vi "USRP_singlecarrierTDMUSRP1.vi"() -> ()   [LabVIEW 2021]
uses:
  <vilib>/addons/Modulation/Analog/controls/Complex Data Waveform.ctl
  <vilib>/Analysis/coordinate.llb/Angle Units.ctl
  <vilib>/Analysis/coordinate.llb/Angle Range (Degree).ctl
  <vilib>/Analysis/coordinate.llb/Wrap Angle (scalar).vi
  system stop.vi
  <vilib>/measure/matone.llb/Extract Single Tone Information 1 Chan (CDB).vi
  <instrlib>/niUSRP/niUSRP Fetch Rx Data (CDB Cluster).vi
  <instrlib>/niUSRP/niUSRP Write Tx Data (CDB Cluster).vi
  <vilib>/addons/Modulation/niAMT.lvlib
  <vilib>/measure/NI_MAPro.lvlib
  <vilib>/Analysis/NI_AAL_Angle.lvlib
panel:
  in  "Tab Control":T1(tab)
  in  "IQ rate Tx":dbl=400000.0 format="%#_6p"
  in  "Tx Gain":dbl format="%#_6f"
  in  "Tx IP":refnum<k15>="192.168.10.2"
  out "coerced IQ rate Tx":dbl=100000.0 format="%#_6p"
  out "coerced carrier frequency Tx":dbl=100000.0 format="%#_6p"
  in  "Rx IP":refnum<k15>="192.168.10.2"
  in  "Rx gain":dbl format="%#_6f"
  in  "Frequency":dbl=10000.0 format="%#_13g"
  in  "Duration":dbl=0.01 format="%#_13g"
  out "coerced IQ rate Rx":dbl=100000.0 format="%#_6p"
  out "coerced carrier frequency Rx":dbl=100000.0 format="%#_6p"
  in  "number of samples":i64=4000
  in  "carrier frequency":dbl=2400000000.0 format="%#_6p"
  in  "Phase in deg":dbl
  out "Counter":dbl
  out "Waveform Graph":dbl[](graph)
  out "Boolean":bool
  out "detected frequency":dbl format="%.2p"
  out "detected Amplitude":dbl format="%.2p"
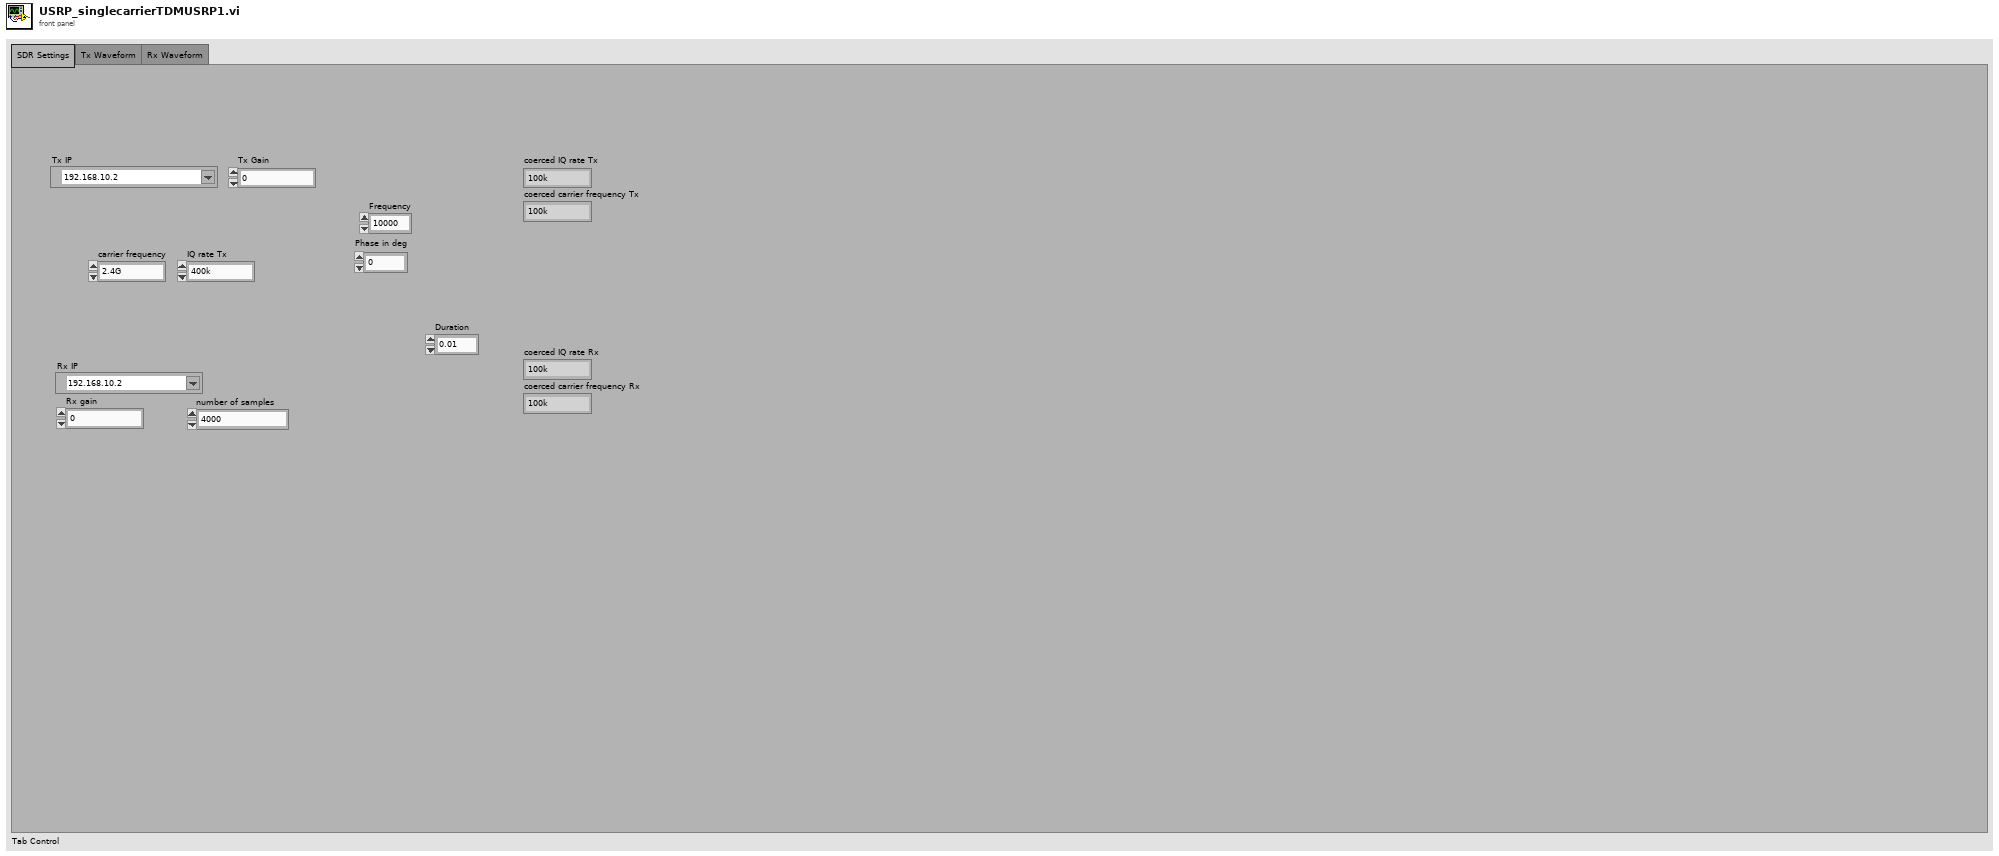
[diagram p1: front panel]
types:
  T1 = enum32{"SDR Settings", "Tx Waveform", "Rx Waveform"}
  T2 = typedef "niAMT.lvlib/Complex Data Waveform.ctl" = cluster{"t0":dbl, "dt":dbl, "Y":cdb[]}
  T3 = typedef "NI_AAL_Angle.lvlib/Angle Range (Degree).ctl" = u16
  T4 = typedef "NI_AAL_Angle.lvlib/Angle Units.ctl" = i32
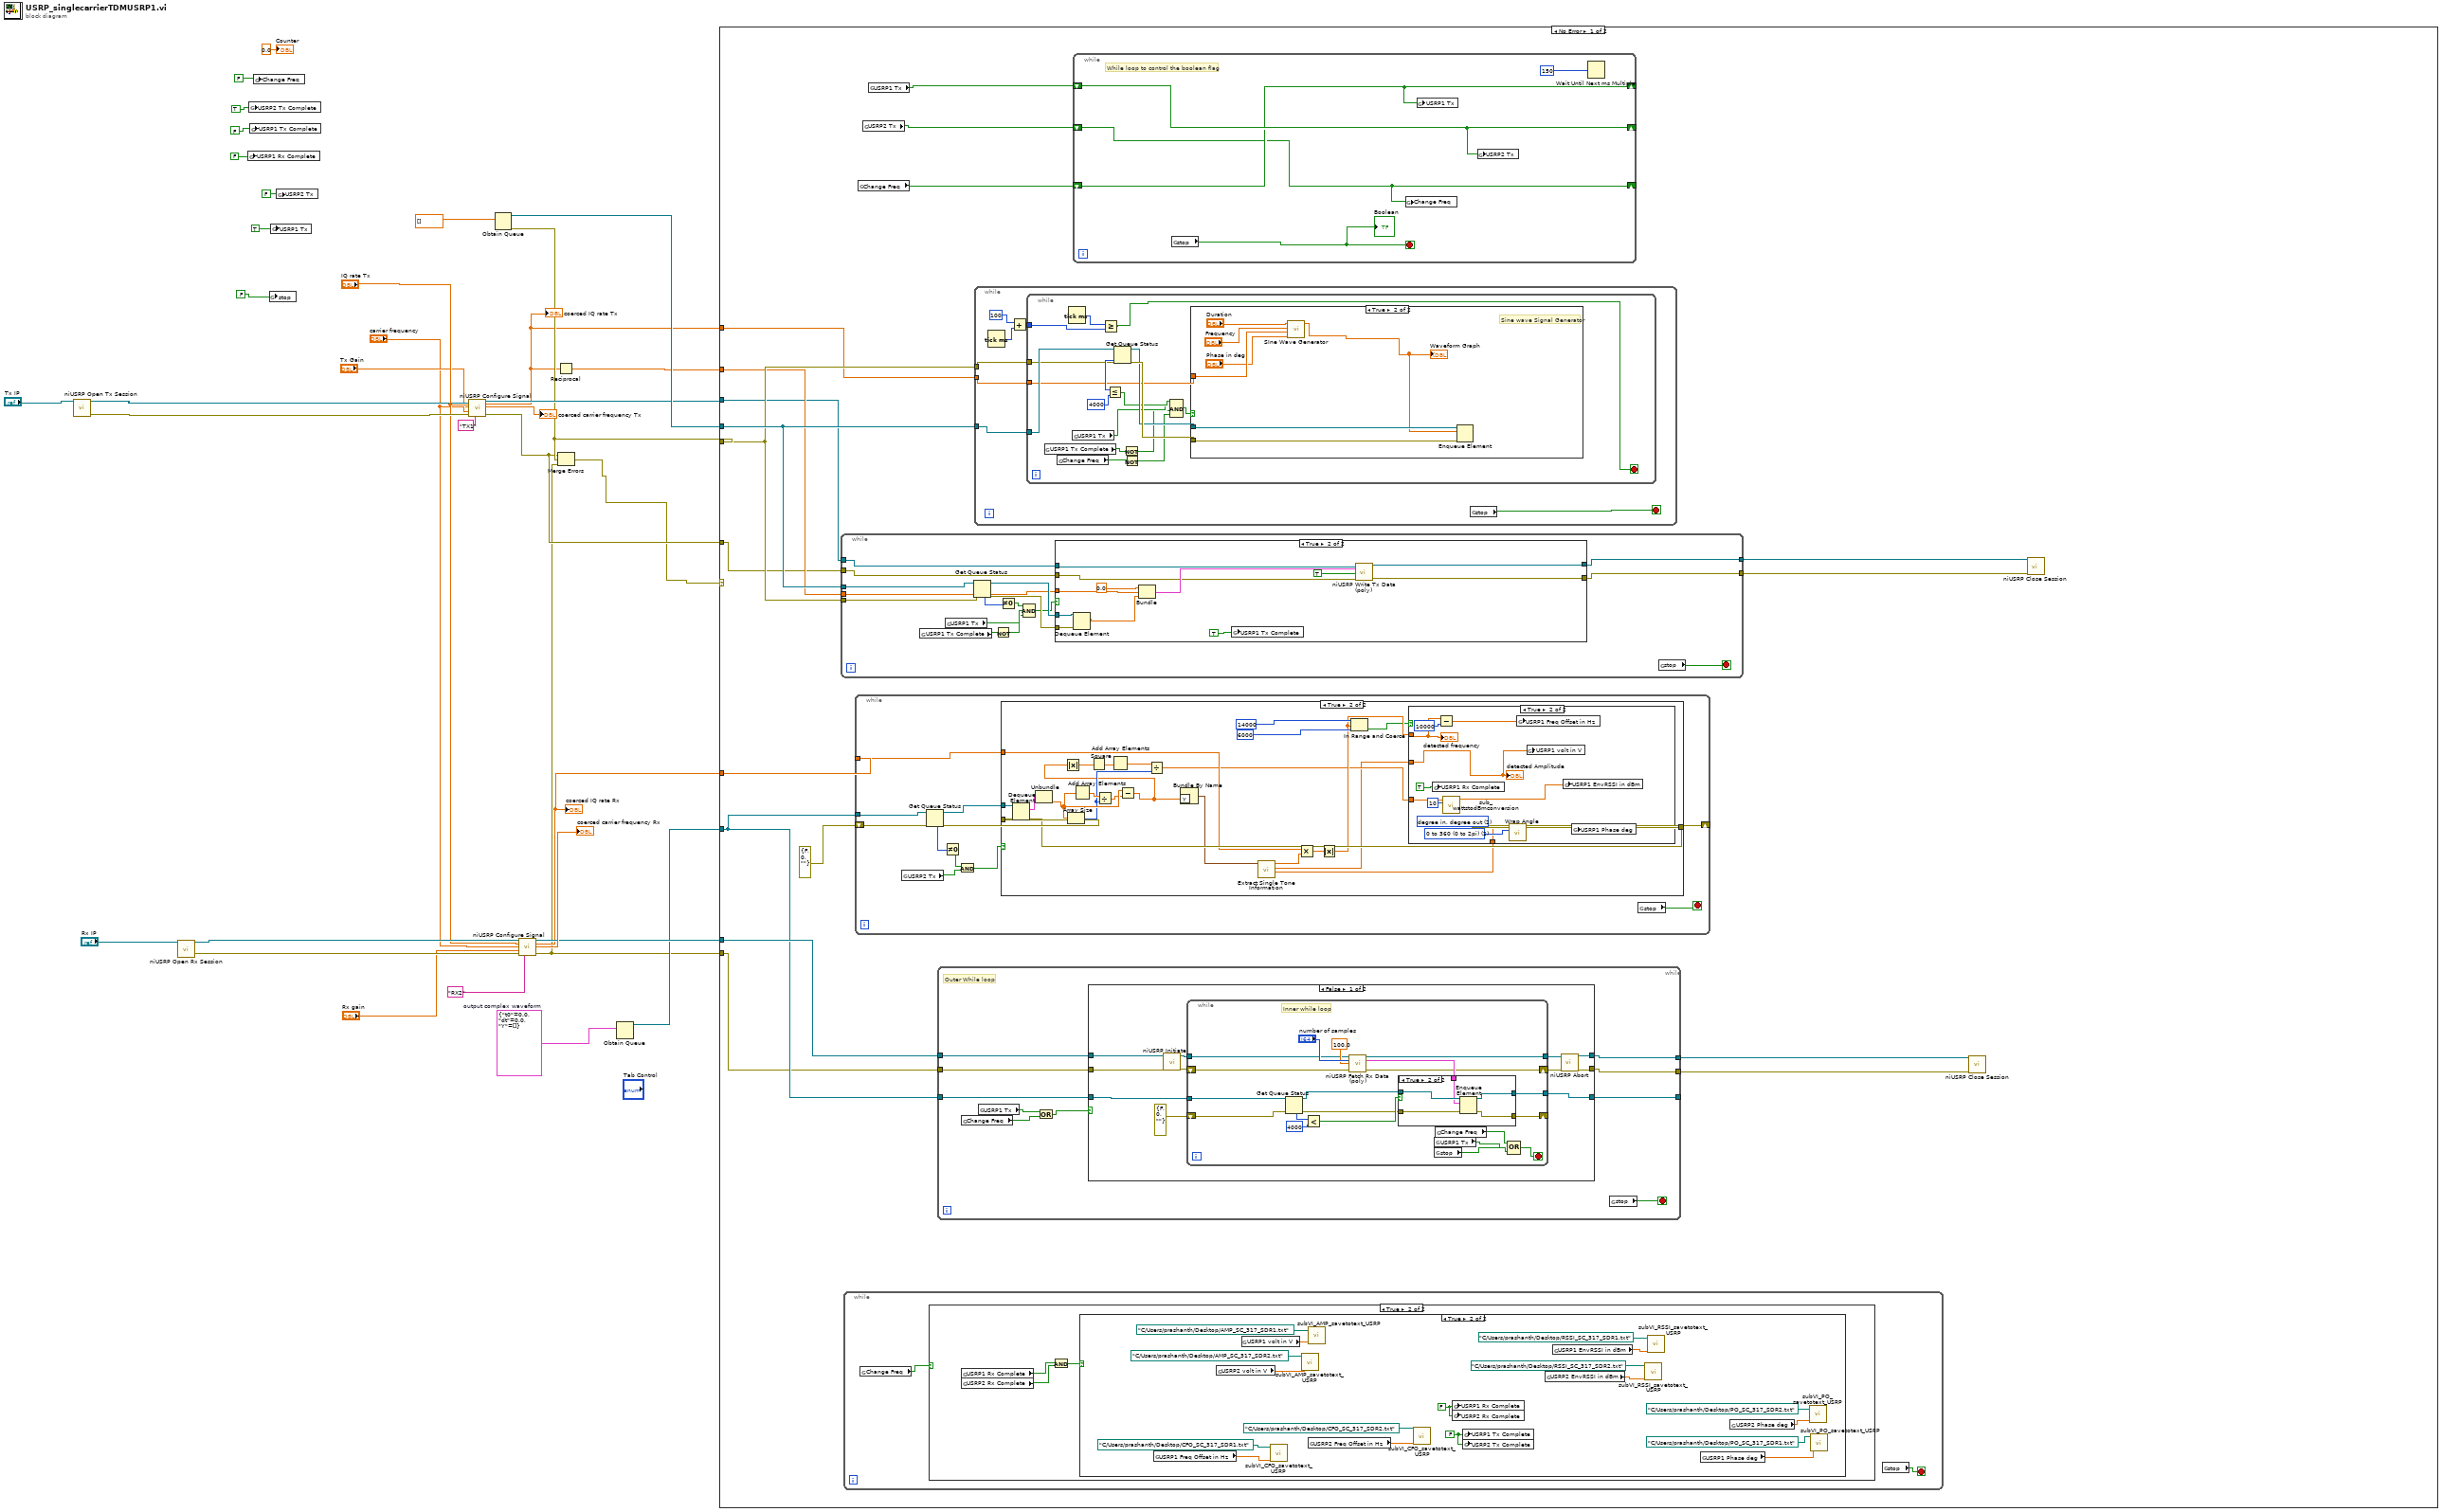
[diagram p0: block diagram]
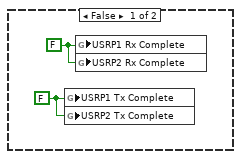
[diagram p3: hidden frame]
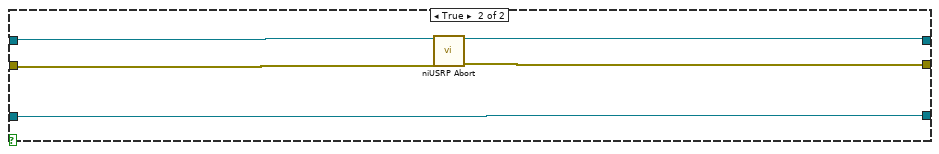
[diagram p6: hidden frame]
diagram:
  w9 = T2 {"t0"=0.0, "dt"=0.0, "Y"=[]}  # output complex waveform
  n1 = call <instrlib>:"niUSRP Open Tx Session.vi"("device names"="Tx IP") -> ("session handle out"=w34:refnum<k15>, "error out"=w33:errorcluster)  [unwired: 13 in]
  n2 = call <instrlib>:"niUSRP Open Rx Session.vi"("device names"="Rx IP") -> ("session handle out"=w31:refnum<k15>, "error out"=w30:errorcluster)  [unwired: 13 in]
  n3 = global write "system stop.vi" "USRP1 Rx Complete"(FALSE) -> ()
  n4 = global write "system stop.vi" "USRP2 Tx Complete"(TRUE) -> ()
  n5 = global write "system stop.vi" "USRP1 Tx Complete"(FALSE) -> ()
  n6 = global write "system stop.vi" "Change Freq"(FALSE) -> ()
  n7 = global write "system stop.vi" "stop"(FALSE) -> ()
  n8 = global write "system stop.vi" "USRP1 Tx"(TRUE) -> ()
  n9 = global write "system stop.vi" "USRP2 Tx"(FALSE) -> ()
  n10 = call <instrlib>:"niUSRP Configure Signal.vi"("session handle"=w34, "IQ rate"="IQ rate Tx", "carrier frequency"="carrier frequency", "gain"="Tx Gain", "error in (no error)"=w33, "active antenna"="TX1") -> ("session handle out"=w16:refnum<k15>, "coerced IQ rate"=w13:dbl, "coerced carrier frequency"=→"coerced carrier frequency Tx":dbl, "error out"=w12:errorcluster)  [unwired: 5 in, 1 out]
  "coerced IQ rate Tx" <- w13
  n11 = Obtain Queue(element data type=dbl[] []) -> (queue out=w17:refnum<queue>, error out=w14:errorcluster)  [unwired: 4 in, 1 out]
  n12 = call <instrlib>:"niUSRP Configure Signal.vi"("session handle"=w31, "IQ rate"="IQ rate Tx", "carrier frequency"="carrier frequency", "gain"="Rx gain", "error in (no error)"=w30, "active antenna"="RX2") -> ("session handle out"=w10:refnum<k15>, "coerced IQ rate"=w7:dbl, "coerced carrier frequency"=→"coerced carrier frequency Rx":dbl, "error out"=w6:errorcluster)  [unwired: 5 in, 1 out]
  "coerced IQ rate Rx" <- w7
  n13 = Reciprocal(x=w13) -> (1/x=w15:dbl)
  n14 = Merge Errors(w12, w14, w6) -> (w4:errorcluster)
  n15 = Obtain Queue(element data type=w9) -> (queue out=w8:refnum<queue>)  [unwired: 4 in, 2 out]
  n16 = case shown="No Error" w4 {
    tunnel: w14 -> [w52 _]
    tunnel: w17 -> [w53 _]
    tunnel: w16 -> [w50 _]
    tunnel: w15 -> [w51 _]
    tunnel: w13 -> [w49 _]
    tunnel: w12 -> [w48 _]
    tunnel: w10 -> [w46 _]
    tunnel: w8 -> [w45 _]
    tunnel: w7 -> [w44 _]
    tunnel: w6 -> [w43 _]
    frame No Error {
      n17 = while {
        tunnel: w52 -> [w227]
        tunnel: w51 -> [w226]
        tunnel: w50 -> [w223]
        tunnel: w48 -> [w222]
        tunnel: [w218] -> w39
        tunnel: [w217] -> w38
        tunnel: w53 -> [w230]
        stop <- w224 stop-if-true
        n18 = global read "system stop.vi" "USRP1 Tx Complete"() -> (w219:bool)
        n19 = global read "system stop.vi" "USRP1 Tx"() -> (w215:bool)
        n20 = Get Queue Status(queue=w230, error in (no error)=w227) -> (queue out=w229:refnum<queue>, error out=w228:errorcluster, # elements in queue=w225:i32)  [unwired: 1 in, 5 out]
        n21 = Not(x=w219) -> (.not. x?=w220:bool)
        n22 = Not Equal To 0?(x=w225) -> (x != 0?=w221:bool)
        n23 = Compound Arithmetic op=AND(w221, w220, w215) -> (w216:bool)
        n24 = case shown="True" w216 {
          tunnel: w229 -> [_ w244]
          tunnel: w228 -> [_ w243]
          tunnel: w226 -> [_ w242]
          tunnel: w223 -> [w232 w235]
          tunnel: w222 -> [w231 w234]
          tunnel: [w232 w238] -> w218
          tunnel: [w231 w236] -> w217
          frame False {
          }
          frame True {
            n25 = Dequeue Element(queue=w244, error in (no error)=w243) -> (element=w233:dbl[])  [unwired: 1 in, 3 out]
            n26 = Bundle(0.0, w242, w233) -> (w241:cluster{dbl, dbl, dbl[]})  [unwired: 1 in]
            n27 = global write "system stop.vi" "USRP1 Tx Complete"(TRUE) -> ()
            n28 = call-poly <instrlib>:"niUSRP Write Tx Data (poly).vi"("session handle"=w235, "data"=w241, "end of data?"=TRUE, "error in (no error)"=w234) -> ("session handle out"=w238:refnum<k15>, "error out"=w236:errorcluster)  [unwired: 10 in]
          }
        }
        n29 = global read "system stop.vi" "stop"() -> (w224:bool)
      }
      n30 = while {
        stop <- w54 stop-if-true
        n31 = global read "system stop.vi" "Change Freq"() -> (w55:bool)
        n32 = case shown="True" w55 {
          frame False {
          }
          frame True {
            n33 = global read "system stop.vi" "USRP1 Rx Complete"() -> (w58:bool)
            n34 = global read "system stop.vi" "USRP2 Rx Complete"() -> (w57:bool)
            n35 = And(x=w58, y=w57) -> (x .and. y?=w56:bool)
            n36 = case shown="True" w56 {
              frame False {
                w60 = FALSE
                w59 = FALSE
                n37 = global write "system stop.vi" "USRP1 Tx Complete"(w60) -> ()
                n38 = global write "system stop.vi" "USRP2 Tx Complete"(w60) -> ()
                n39 = global write "system stop.vi" "USRP1 Rx Complete"(w59) -> ()
                n40 = global write "system stop.vi" "USRP2 Rx Complete"(w59) -> ()
              }
              frame True {
                w78 = FALSE
                w77 = FALSE
                n41 = global read "system stop.vi" "USRP1 Freq Offset in Hz"() -> (w71:dbl)
                n42 = global read "system stop.vi" "USRP2 volt in V"() -> (w74:dbl)
                n43 = global read "system stop.vi" "USRP1 volt in V"() -> (w75:dbl)
                n44 = call "subVI_CFO_savetotext_USRP.vi"("RSSI"=w71, "file path (dialog if empty)"=path "C:/Users/prashanth/Desktop/CFO_SC_317_SDR1.txt") -> ()  [unwired: 10 in]
                n45 = call "subVI_AMP_savetotext_USRP.vi"("RSSI"=w74, "file path (dialog if empty)"=path "C:/Users/prashanth/Desktop/AMP_SC_317_SDR2.txt") -> ()  [unwired: 10 in]
                n46 = call "subVI_AMP_savetotext_USRP.vi"("RSSI"=w75, "file path (dialog if empty)"=path "C:/Users/prashanth/Desktop/AMP_SC_317_SDR1.txt") -> ()  [unwired: 10 in]
                n47 = global read "system stop.vi" "USRP2 Freq Offset in Hz"() -> (w69:dbl)
                n48 = call "subVI_CFO_savetotext_USRP.vi"("RSSI"=w69, "file path (dialog if empty)"=path "C:/Users/prashanth/Desktop/CFO_SC_317_SDR2.txt") -> ()  [unwired: 10 in]
                n49 = global write "system stop.vi" "USRP1 Rx Complete"(w77) -> ()
                n50 = global write "system stop.vi" "USRP2 Rx Complete"(w77) -> ()
                n51 = global write "system stop.vi" "USRP1 Tx Complete"(w78) -> ()
                n52 = global write "system stop.vi" "USRP2 Tx Complete"(w78) -> ()
                n53 = global read "system stop.vi" "USRP2 EnvRSSI in dBm"() -> (w67:dbl)
                n54 = global read "system stop.vi" "USRP1 EnvRSSI in dBm"() -> (w65:dbl)
                n55 = call "subVI_RSSI_savetotext_USRP.vi"("RSSI"=w67, "file path (dialog if empty)"=path "C:/Users/prashanth/Desktop/RSSI_SC_317_SDR2.txt") -> ()  [unwired: 10 in]
                n56 = call "subVI_RSSI_savetotext_USRP.vi"("RSSI"=w65, "file path (dialog if empty)"=path "C:/Users/prashanth/Desktop/RSSI_SC_317_SDR1.txt") -> ()  [unwired: 10 in]
                n57 = global read "system stop.vi" "USRP1 Phase deg"() -> (w63:dbl)
                n58 = global read "system stop.vi" "USRP2 Phase deg"() -> (w61:dbl)
                n59 = call "subVI_PO_savetotext_USRP.vi"("RSSI"=w61, "file path (dialog if empty)"=path "C:/Users/prashanth/Desktop/PO_SC_317_SDR2.txt") -> ()  [unwired: 10 in]
                n60 = call "subVI_PO_savetotext_USRP.vi"("RSSI"=w63, "file path (dialog if empty)"=path "C:/Users/prashanth/Desktop/PO_SC_317_SDR1.txt") -> ()  [unwired: 10 in]
              }
            }
          }
        }
        n61 = global read "system stop.vi" "stop"() -> (w54:bool)
      }
      n62 = while {
        tunnel: w45 -> [w175]
        shift-right: [w173] -> _
        shift-left: errorcluster {"status"=FALSE, "code"=0, "source"=""} ("error in (no error)") -> [w174]
        tunnel: w44 -> [w172]
        stop <- w171 stop-if-true
        n63 = global read "system stop.vi" "USRP2 Tx"() -> (w170:bool)
        n64 = Get Queue Status(queue=w175, error in (no error)=w174) -> (queue out=w177:refnum<queue>, error out=w176:errorcluster, # elements in queue=w178:i32)  [unwired: 1 in, 5 out]
        n65 = Not Equal To 0?(x=w178) -> (x != 0?=w169:bool)
        n66 = And(x=w169, y=w170) -> (x .and. y?=w168:bool)
        n67 = case shown="True" w168 {
          tunnel: w177 -> [_ w202]
          tunnel: w176 -> [w179 w201]
          tunnel: [w179 w196] -> w173
          tunnel: w172 -> [_ w194]
          frame False {
          }
          frame True {
            n68 = Dequeue Element(queue=w202, error in (no error)=w201) -> (element=w200:T2, error out=w196:errorcluster)  [unwired: 1 in, 2 out]
            n69 = Unbundle(w200) -> ("Y"=w191:cdb[])  [unwired: 2 out]
            n70 = Array Size(array=w191) -> (size(s)=w188:i32)
            n71 = Add Array Elements(numeric array=w191) -> (sum=w199:cdb)
            n72 = Divide(x=w199, y=w188) -> (x/y=w189:cdb)
            n73 = Subtract(x=w191, y=w189) -> (x-y=w183:cdb[])
            n74 = Absolute Value(x=w183) -> (abs(x)=w190:dbl[])
            n75 = Square(x=w190) -> (x^2=w187:dbl[])
            n76 = Add Array Elements(numeric array=w187) -> (sum=w186:dbl)
            n77 = Divide(x=w186, y=w188) -> (x/y=w185:dbl)
            n78 = Bundle By Name("Y"=w183) -> (w180:waveform(cdb))  [unwired: 1 in]
            n79 = call-poly <vilib>:"Extract Single Tone Information.vi"("time signal in"=w180) -> ("detected phase (deg)"=w184:dbl, "detected amplitude"=w182:dbl, "detected frequency"=w195:dbl)  [unwired: 5 in, 3 out]
            n80 = Multiply(x=w194, y=w195) -> (x*y=w193:dbl)
            n81 = Absolute Value(x=w193) -> (abs(x)=w192:dbl)
            n82 = In Range and Coerce(upper limit=14000, x=w192, lower limit=6000) -> (In Range?=w181:bool)  [unwired: 1 out]
            n83 = case shown="True" w181 {
              tunnel: w192 -> [_ w213]
              tunnel: w182 -> [_ w203]
              tunnel: w185 -> [_ w210]
              tunnel: w184 -> [_ w205]
              frame False {
              }
              frame True {
                w207 = T3 2 items=["none", "-180 to 180 (-pi to pi)", "0 to 360 (0 to 2pi)"] ("angle range")
                w208 = T4 2 items=["radian in, radian out", "radian in, degree out", "degree in, degree out", "degree in, radian out"] ("angle units")
                n84 = global write "system stop.vi" "USRP1 Rx Complete"(TRUE) -> ()
                n85 = Subtract(x=w213, y=10000) -> (x-y=w211:dbl)
                n86 = call "sub_wattstodBmconversion.vi"("Amp or Power"=10, "detected amplitude"=w210) -> ("Numeric"=w209:dbl)  [unwired: 9 in]
                n87 = call-poly <vilib>:"Wrap Angle.vi"("angle units"=w208, "angle range"=w207, "angle in"=w205) -> ("angle out"=w206:dbl)  [unwired: 7 in, 1 out]
                n88 = global write "system stop.vi" "USRP1 Freq Offset in Hz"(w211) -> ()
                n89 = global write "system stop.vi" "USRP1 volt in V"(w203) -> ()
                n90 = global write "system stop.vi" "USRP1 EnvRSSI in dBm"(w209) -> ()
                n91 = global write "system stop.vi" "USRP1 Phase deg"(w206) -> ()
                "detected frequency" <- w213
                "detected Amplitude" <- w203
              }
            }
          }
        }
        n92 = global read "system stop.vi" "stop"() -> (w171:bool)
      }
      n93 = global read "system stop.vi" "Change Freq"() -> (w41:bool)
      n94 = global read "system stop.vi" "USRP2 Tx"() -> (w40:bool)
      n95 = global read "system stop.vi" "USRP1 Tx"() -> (w42:bool)
      n96 = while {
        tunnel: w46 -> [w122]
        tunnel: w43 -> [w121]
        tunnel: [w116] -> w37
        tunnel: [w115] -> w36
        tunnel: w45 -> [w124]
        tunnel: [w120] -> _
        stop <- w123 stop-if-true
        # "Outer While loop"
        n97 = global read "system stop.vi" "Change Freq"() -> (w117:bool)
        n98 = global read "system stop.vi" "USRP1 Tx"() -> (w118:bool)
        n99 = Compound Arithmetic op=OR(w118, w117) -> (w119:bool)
        n100 = case shown="False" w119 {
          tunnel: w122 -> [w127 w167]
          tunnel: w124 -> [w135 w163]
          tunnel: w121 -> [w126 w165]
          tunnel: [w130 w166] -> w116
          tunnel: [w129 w164] -> w115
          tunnel: [w125 w163] -> w120
          frame False {
            n101 = call <instrlib>:"niUSRP Initiate.vi"("session handle"=w127, "error in (no error)"=w126) -> ("session handle out"=w133:refnum<k15>, "error out"=w132:errorcluster)  [unwired: 12 in]
            n102 = while {
              tunnel: w135 -> [w155]
              shift-right: [w139] -> w128
              shift-left: w132 -> [w141]
              shift-right: [w154] -> _
              shift-left: errorcluster {"status"=FALSE, "code"=0, "source"=""} ("error in (no error)") -> [w153]
              tunnel: w133 -> [w142]
              tunnel: [w140] -> w131
              tunnel: [w136] -> w125
              stop <- w145 stop-if-true
              # "Inner while loop"
              n103 = Get Queue Status(queue=w155, error in (no error)=w153) -> (queue out=w148:refnum<queue>, error out=w149:errorcluster, # elements in queue=w152:i32)  [unwired: 1 in, 5 out]
              n104 = Less?(x=w152, y=4000) -> (x < y?=w150:bool)
              n105 = call-poly <instrlib>:"niUSRP Fetch Rx Data (poly).vi"("session handle"=w142, "number of samples"="number of samples", "timeout"=100.0, "error in (no error)"=w141) -> ("session handle out"=w140:refnum<k15>, "data"=w146:cluster{"t0":dbl, "dt":dbl, "Y":cdb[]}, "error out"=w139:errorcluster)  [unwired: 8 in, 1 out]
              n106 = case shown="True" w150 {
                tunnel: w149 -> [w157 w162]
                tunnel: w148 -> [w156 w161]
                tunnel: w146 -> [_ w160]
                tunnel: [w157 w159] -> w154
                tunnel: [w156 w158] -> w136
                frame False {
                }
                frame True {
                  n107 = Enqueue Element(queue=w161, element=w160, error in (no error)=w162) -> (queue out=w158:refnum<queue>, error out=w159:errorcluster)  [unwired: 1 in, 1 out]
                }
              }
              n108 = global read "system stop.vi" "USRP1 Tx"() -> (w138:bool)
              n109 = global read "system stop.vi" "stop"() -> (w144:bool)
              n110 = global read "system stop.vi" "Change Freq"() -> (w137:bool)
              n111 = Compound Arithmetic op=OR(w137, w138, w144) -> (w145:bool)
            }
            n112 = call <instrlib>:"niUSRP Abort.vi"("session handle"=w131, "error in (no error)"=w128) -> ("session handle out"=w130:refnum<k15>, "error out"=w129:errorcluster)  [unwired: 12 in]
          }
          frame True {
            n113 = call <instrlib>:"niUSRP Abort.vi"("session handle"=w167, "error in (no error)"=w165) -> ("session handle out"=w166:refnum<k15>, "error out"=w164:errorcluster)  [unwired: 12 in]
          }
        }
        n114 = global read "system stop.vi" "stop"() -> (w123:bool)
      }
      n115 = while {
        tunnel: w52 -> [w89]
        tunnel: w49 -> [w88]
        tunnel: w53 -> [w90]
        stop <- w84 stop-if-true
        n116 = Tick Count (ms)() -> (millisecond timer value=w86:u32)
        n117 = Add(x=100, y=w86) -> (x+y=w85:u32)
        n118 = while {
          tunnel: w89 -> [w102]
          tunnel: w88 -> [w101]
          tunnel: w85 -> [w96]
          tunnel: w90 -> [w103]
          stop <- w92 stop-if-true
          n119 = global read "system stop.vi" "USRP1 Tx Complete"() -> (w94:bool)
          n120 = global read "system stop.vi" "Change Freq"() -> (w93:bool)
          n121 = Tick Count (ms)() -> (millisecond timer value=w97:u32)
          n122 = global read "system stop.vi" "USRP1 Tx"() -> (w99:bool)
          n123 = Greater Or Equal?(x=w97, y=w96) -> (x >= y?=w92:bool)
          n124 = Get Queue Status(queue=w103, error in (no error)=w102) -> (queue out=w104:refnum<queue>, error out=w105:errorcluster, # elements in queue=w107:i32)  [unwired: 1 in, 5 out]
          n125 = Less Or Equal?(x=w107, y=4000) -> (x <= y?=w100:bool)
          n126 = Not(x=w94) -> (.not. x?=w95:bool)
          n127 = Not(x=w93) -> (.not. x?=w91:bool)
          n128 = Compound Arithmetic op=AND(w100, w99, w95, w91) -> (w98:bool)
          n129 = case shown="True" w98 {
            tunnel: w105 -> [_ w114]
            tunnel: w104 -> [_ w113]
            tunnel: w101 -> [_ w110]
            frame False {
            }
            frame True {
              # "Sine wave Signal Generator"
              n130 = call "SIne Wave Generator.vi"("Phase in deg"="Phase in deg", "Sampling rate"=w110, "Frequency"="Frequency", "Duration"="Duration") -> ("Array"=w108:dbl[])  [unwired: 6 in, 1 out]
              "Waveform Graph" <- w108
              n131 = Enqueue Element(queue=w113, element=w108, error in (no error)=w114) -> ()  [unwired: 1 in, 3 out]
            }
          }
        }
        n132 = global read "system stop.vi" "stop"() -> (w84:bool)
      }
      n133 = while {
        shift-right: [w81] -> _
        shift-left: w42 -> [w83]
        shift-right: [w83] -> _
        shift-left: w40 -> [w80]
        shift-right: [w80] -> _
        shift-left: w41 -> [w81]
        stop <- w82 stop-if-true
        # "While loop to control the boolean flag"
        n134 = global read "system stop.vi" "stop"() -> (w82:bool)
        "Boolean" <- w82
        n135 = global write "system stop.vi" "Change Freq"(w80) -> ()
        n136 = global write "system stop.vi" "USRP1 Tx"(w81) -> ()
        n137 = global write "system stop.vi" "USRP2 Tx"(w83) -> ()
        n138 = Wait Until Next ms Multiple(millisecond multiple=150) -> ()  [unwired: 1 out]
      }
      n139 = call <instrlib>:"niUSRP Close Session.vi"("session handle"=w37, "error in (no error)"=w36) -> ()  [unwired: 13 in, 1 out]
      n140 = call <instrlib>:"niUSRP Close Session.vi"("session handle"=w39, "error in (no error)"=w38) -> ()  [unwired: 13 in, 1 out]
    }
    frame Error {
    }
  }
  "Counter" <- 0.0 ("Counter")
